vi "SubVI_Yellow Spot #.vi"(5 "»Ö­È":i16, 7 "Image Register Name":string="untitled", 8 "Error In":errorcluster, 9 "B":u8[][](array[numeric]), 10 "G":u8[][](array[numeric]), 11 "R":u8[][](array[numeric])) -> (0 "Error Out":errorcluster, 3 "Image Dst Out":T1)   [LabVIEW 2013]
uses:
  <vilib>/vision/Image Controls.llb/IMAQ Image.ctl
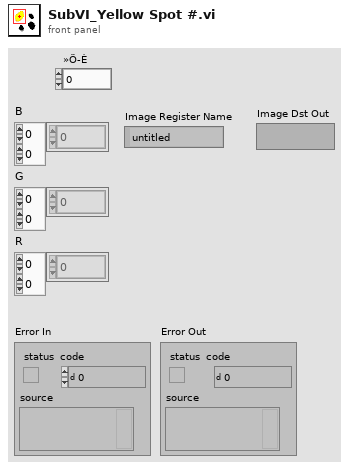
[diagram p1: front panel]
types:
  T1 = typedef "IMAQ Image.ctl" = refnum<image>
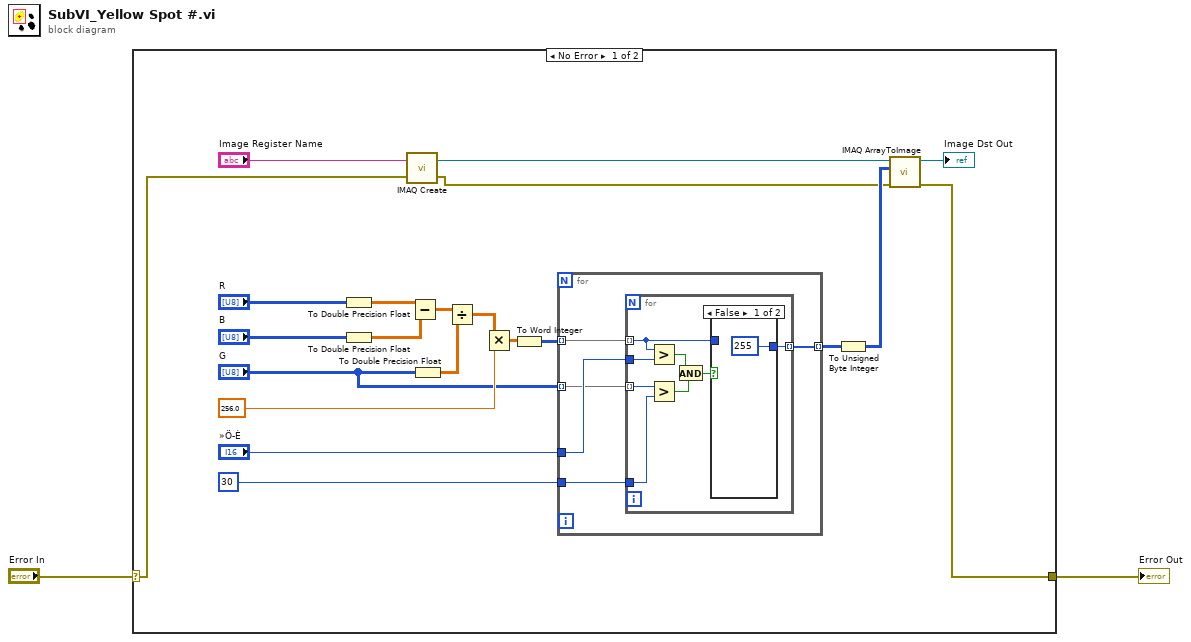
[diagram p0: block diagram]
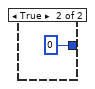
[diagram p2: hidden frame]
diagram:
  n1 = case shown="No Error" "Error In" {
    selector: "Error In" -> [w5 w39]
    tunnel: [w3 w39] -> w1
    frame No Error {
      n2 = To Double Precision Float(number="R") -> (double precision float=w16:dbl[][])
      n3 = To Double Precision Float(number="B") -> (double precision float=w14:dbl[][])
      n4 = call "IMAQ Create"("Image Name"="Image Register Name", "error in (no error)"=w5) -> ("New Image"=w6:T1, "error out"=w4:errorcluster)  [unwired: 3 in]
      n5 = Subtract(x=w16, y=w14) -> (x-y=w15:dbl[][])
      n6 = To Double Precision Float(number="G") -> (double precision float=w19:dbl[][])
      n7 = Divide(x=w15, y=w19) -> (x/y=w17:dbl[][])
      n8 = Multiply(x=w17, y=256.0) -> (x*y=w13:dbl[][])
      n9 = To Word Integer(number=w13) -> (16bit integer=w12:i16[][])
      n10 = for {
        tunnel: w12 -> [w28] mode=indexing
        tunnel: "»Ö­È" -> [w27]
        tunnel: [w26] -> w22 mode=indexing
        tunnel: "G" -> [w25] mode=indexing
        tunnel: u8 30 -> [w24]
        n11 = for {
          tunnel: w28 -> [w35] mode=indexing
          tunnel: w27 -> [w36]
          tunnel: [w34] -> w26 mode=indexing
          tunnel: w25 -> [w33] mode=indexing
          tunnel: w24 -> [w32]
          n12 = Greater?(x=w35, y=w36) -> (0:w31:bool)
          n13 = Greater?(x=w33, y=w32) -> (0:w30:bool)
          n14 = And(x=w31, y=w30) -> (x .and. y?=w29:bool)
          n15 = case shown="False" w29 {
            tunnel: w35 -> [_ _]
            tunnel: [i16 255 ("element") i16 0 ("element")] -> w34
            frame False {
            }
            frame True {
            }
          }
        }
      }
      n16 = To Unsigned Byte Integer(number=w22) -> (unsigned 8bit integer=w21:u8[][])
      n17 = call "IMAQ ArrayToImage"("error in (no error)"=w4, "Image Pixels (U8)"=w21, "Image"=w6) -> ("error out"=w3:errorcluster, "Image Out"=→"Image Dst Out":T1)  [unwired: 7 in]
    }
    frame Error {
    }
  }
  "Error Out" <- w1
